vi "test-trajectory-generator-initial-config.vi"() -> (3 "traj_config":T1 {"End Velocity" format="%20.4f"; "StartVelocity" format="%20.4f"; "Max Acceleration" format="%20.4f"; "MaxVelocity" format="%20.4f"})   [LabVIEW 2019]
uses:
  <vilib>/Rock Robotics/WPI/ThirdParty/JAS_Junk/TrajLib/TRAJ_CONFIG.ctl
  <vilib>/Rock Robotics/WPI/ThirdParty/JAS_Junk/TrajLib/Trajectory_Library.lvlib
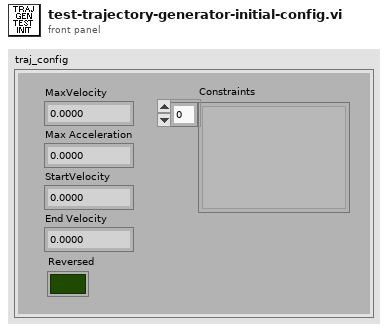
[diagram p1: front panel]
types:
  T1 = typedef "Trajectory_Library.lvlib/TRAJ_CONFIG.ctl" = cluster{"MaxVelocity":dbl, "Max Acceleration":dbl, "StartVelocity":dbl, "End Velocity":dbl, "Reversed":bool, "Constraints":variant[]}
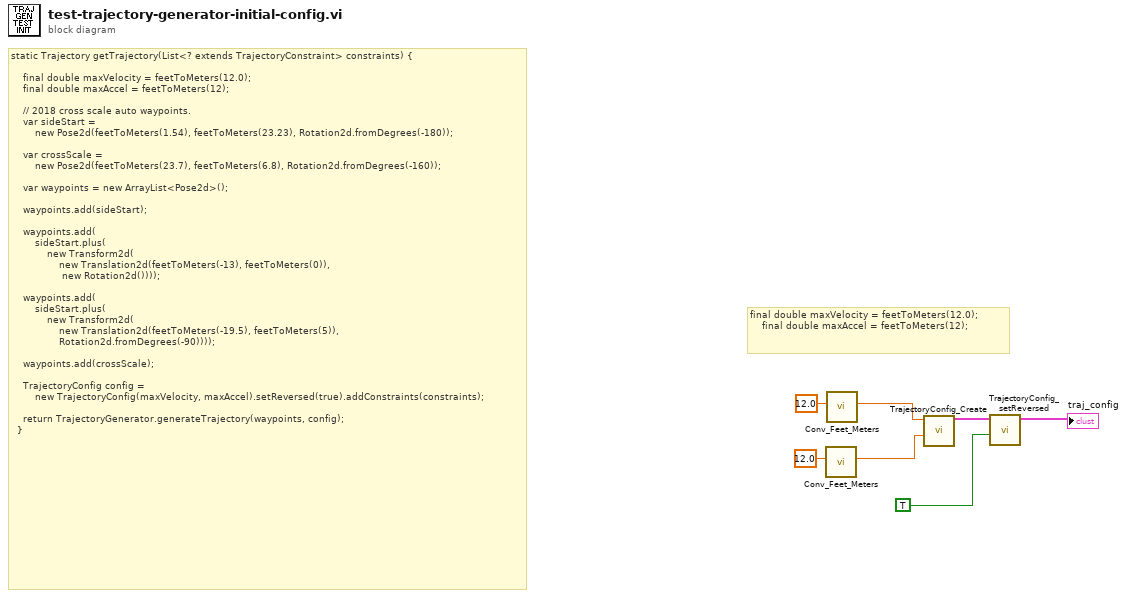
[diagram p0: block diagram]
diagram:
  # "final double maxVelocity = feetToMeters(12.0);\n    final double maxAccel = feetToMeters(12);"
  # "static Trajectory getTrajectory(List<? extends TrajectoryConstraint> constraints) {\n\n    final double maxVelocity = feetToMeters(12.0);\n    final double maxAccel = feetToMeters(12);\n\n    // 2018 cross scale auto waypoints.\n    var sideStart =\n        new Pose2d(feetToMeters(1.54), feetToMeters(23.23), Rotation2d.fromDegrees(-180));\n\n    var crossScale =\n        new Pose2d(feetToMeters(23.7), feetToMeters(6.8), Rotation2d.fromDegrees(-160));\n\n    var waypoints = new ArrayList<Pose2d>();\n\n    waypoints.add(sideStart);\n\n    waypoints.add(\n        sideStart.plus(\n            new Transform2d(\n                new Translation2d(feetToMeters(-13), feetToMeters(0)), \n                 new Rotation2d())));\n\n    waypoints.add(\n        sideStart.plus(\n            new Transform2d(\n                new Translation2d(feetToMeters(-19.5), feetToMeters(5)),\n                Rotation2d.fromDegrees(-90))));\n\n    waypoints.add(crossScale);\n\n    TrajectoryConfig config =\n        new TrajectoryConfig(maxVelocity, maxAccel).setReversed(true).addConstraints(constraints);\n\n    return TrajectoryGenerator.generateTrajectory(waypoints, config);\n  }"
  n1 = call <vilib>:"Conv_Feet_Meters.vi"("Feet"=12.0) -> ("Meters"=w4:dbl)  [unwired: 10 in]
  n2 = call <vilib>:"Conv_Feet_Meters.vi"("Feet"=12.0) -> ("Meters"=w5:dbl)  [unwired: 10 in]
  n3 = call <vilib>:"TrajectoryConfig_Create.vi"("MaxAcceleration"=w4, "MaxVelocity"=w5) -> ("TRAJECTORY_CONFIG"=w3:T1)  [unwired: 9 in]
  n4 = call <vilib>:"TrajectoryConfig_setReversed.vi"("Reversed"=TRUE, "inTRAJECTORY_CONFIG"=w3) -> ("outTRAJECTORY_CONFIG"=→"traj_config":T1)  [unwired: 9 in]
